vi "globals-engine.vi"() -> ()   [LabVIEW 2024]
uses:
  controls/state-engine.ctl
  controls/type.eng.settings.ctl
  controls/state-logger.ctl
  controls/UiNutritionPanel.ctl
  controls/UiScheduleTimestamp.ctl
  controls/pbr-conf.ctl
  controls/irr-panel.ctl
  controls/enum-com-log.ctl
  controls/enum-q-sched.ctl
panel:
  in  "Q-Sched":refnum<queue>
  out "Q-Com":refnum<queue>
  in  "IRR Params":T1={"Day Time"={"Sunset"=timestamp(0 s since 1904-01-01), "Sunrise"=timestamp(0 s since 1904-01-01)}, "timeLimits"={"Irrigation"=0.0, "Nut./Water"=0.0}, "Calculated Timing"={"Irrigation Timeout"=timestamp(0 s since 1904-01-01), "Nutrients Timeout"=timestamp(0 s since 1904-01-01)}, "Irr Dosing Time"={"Nutrients"=0, "Water"=0, "Wash"=0}, "UV Limit "=0.0, "Dose Table"=[{"Enable"=FALSE, "output"="IRR_SEC1"}, {"Enable"=FALSE, "output"="IRR_SEC2"}, {"Enable"=FALSE, "output"="IRR_SEC3"}, {"Enable"=FALSE, "output"="IRR_SEC4"}, {"Enable"=FALSE, "output"="IRR_SEC5"}, {"Enable"=FALSE, "output"="IRR_SEC6"}], "Last Iteration"=timestamp(0 s since 1904-01-01), "UV Reduction Status"=FALSE, "UV Reduction"=0} {"UV Reduction" max=99 step=1 format="%d [%%]"; "timeLimits"."Nut./Water" format="%02.2f [hr]"; "timeLimits"."Irrigation" format="%02.2f [hr]"; "Day Time"."Sunrise" format="%<%H:%M:%S>T"; "Day Time"."Sunset" format="%<%H:%M:%S>T"; "Calculated Timing"."Nutrients Timeout" format="%<%H:%M:%S>T"; "Calculated Timing"."Irrigation Timeout" format="%<%H:%M:%S>T"; "UV Limit" format="%#.1p [J/m2]"; "Irr Dosing Time"."Wash" format="%d [s]"; "Irr Dosing Time"."Water" format="%d [s]"; "Irr Dosing Time"."Nutrients" format="%d [s]"; "Last Iteration" format="%<%X %x>T"}
  in  "PBRconf":cluster{"units":T2[]} {"units"."Main"."DailyActivityHours"."Begin Time" format="ON:    %<%H:%M>T"; "units"."Main"."DailyActivityHours"."End Time" format="OFF:    %<%H:%M>T"; "units"."Main"."WashTimes"."Out" format="Wash out: %d [sec]"; "units"."Main"."WashTimes"."In" format="Wash in: %d [sec]"}
  in  "NutritionConfiguration":T4[](array[typedef]) {"ORP Dosing"."MIX Limit" format="%d [s]"; "ORP Dosing"."MIX Dose" format="%d [s]"; "PH Dosing"."ACID Limit" format="%d [s]"; "PH Dosing"."BASE Limit" format="%d [s]"; "PH Dosing"."ACID Dose" format="%d [s]"; "PH Dosing"."BASE Dose" format="%d [s]"; "EC Dosing"."BETA2 Limit" format="%d [s]"; "EC Dosing"."ALFA2 Limit" format="%d [s]"; "EC Dosing"."ALFA2 Dose" format="%d [s]"; "EC Dosing"."BETA2 Dose" format="%d [s]"; "EC Dosing"."BETA1 Limit" format="%d [s]"; "EC Dosing"."ALFA1 Limit" format="%d [s]"; "EC Dosing"."ALFA1 Dose" format="%d [s]"; "EC Dosing"."BETA1 Dose" format="%d [s]"; "Main"."DailyActivityHours"."Begin Time" format="ON:    %<%H:%M>T"; "Main"."DailyActivityHours"."End Time" format="OFF:    %<%H:%M>T"; "Main"."WashTimes"."Out" format="Wash out: %d [sec]"; "Main"."WashTimes"."In" format="Wash in: %d [sec]"; "Water Dosing"."Water Limit" format="%d [s]"; "Water Dosing"."Water Dose" format="%d [s]"}
  out "STOP":bool
  in  "Q-Log":refnum<queue>
  in  "NUTRITION_RANGES":T5 {"ALARM"."HIGH" format="%#_13g"; "ALARM"."LOW" format="%#_13g"; "NORMAL"."HIGH" format="%#_13g"; "NORMAL"."LOW" format="%#_13g"}
  in  "ProjectSettings":T6={"Project Name"="Yogiland", "Latitude"=0.0, "Longitude"=0.0, "TimeZone"=0, "userName"="Yogiland"}
  in  "Procedure(pre)":variant[](array[variant])=[variant("procCLK"=variant(dbl 3802946268.2064614), "procIndex"=variant(dbl 2.0), "procIsRunning"=variant(bool TRUE), "procLabel"=variant(string "blink-2"), "procRegisterNumeric"=variant(dbl 3802946266.867457), "procReport"=variant(string "blink-2:3802946268,2>>2,_DELAY_COMPARE,1.3/2.0,STAY"), "procReportPast"=variant(string "blink-2:3802946268,2>>2,_DELAY_COMPARE,1.3/2.0,STAY")), variant("stepFunction"=variant(enum16{"__NO-OP", "_DELAY_LOAD", "_DELAY_COMPARE", "_COMPARE", "_JUMP", "_FINISH", "CLK_COMPARE", "PROC_START", "PROC_STOP", "PROC_ISRUN_COMPARE", "PROC_ISRUN_LOAD", "_IO_READ_IN", "_IO_WRITE_DOUT", "_IO_COMPARE", "Q_OPEN", "Q_WRITE", "Q_READ"} enum."_IO_WRITE_DOUT"), "stepIoPointer"=variant(string "dout2"), "stepIoState(str)"=variant(string "1:1"), "stepLabel"=variant(string "loop"), "stepPath"=variant(string "")), variant("stepFunction"=variant(enum16{"__NO-OP", "_DELAY_LOAD", "_DELAY_COMPARE", "_COMPARE", "_JUMP", "_FINISH", "CLK_COMPARE", "PROC_START", "PROC_STOP", "PROC_ISRUN_COMPARE", "PROC_ISRUN_LOAD", "_IO_READ_IN", "_IO_WRITE_DOUT", "_IO_COMPARE", "Q_OPEN", "Q_WRITE", "Q_READ"} enum."_DELAY_LOAD"), "stepLabel"=variant(string "")), variant("stepFunction"=variant(enum16{"__NO-OP", "_DELAY_LOAD", "_DELAY_COMPARE", "_COMPARE", "_JUMP", "_FINISH", "CLK_COMPARE", "PROC_START", "PROC_STOP", "PROC_ISRUN_COMPARE", "PROC_ISRUN_LOAD", "_IO_READ_IN", "_IO_WRITE_DOUT", "_IO_COMPARE", "Q_OPEN", "Q_WRITE", "Q_READ"} enum."_DELAY_COMPARE"), "stepSetpoint"=variant(cluster{"comparison":string, "Y":dbl} {"comparison"="", "Y"=2.0})), variant("stepFunction"=variant(enum16{"__NO-OP", "_DELAY_LOAD", "_DELAY_COMPARE", "_COMPARE", "_JUMP", "_FINISH", "CLK_COMPARE", "PROC_START", "PROC_STOP", "PROC_ISRUN_COMPARE", "PROC_ISRUN_LOAD", "_IO_READ_IN", "_IO_WRITE_DOUT", "_IO_COMPARE", "Q_OPEN", "Q_WRITE", "Q_READ"} enum."_JUMP"), "stepLabel"=variant(string ""), "stepPointer"=variant(string "loop"))]
  in  "Q-Eng":refnum<queue>
  out "VisaSimulator":bool
  in  "Environment":string
  in  "VISA":refnum<visa-resource-name>
  in  "steps":variant
  in  "stepElemet":variant
  in  "procElement":variant
  # "Water"
  # "EC"
  # "PH"
  # "ORP"
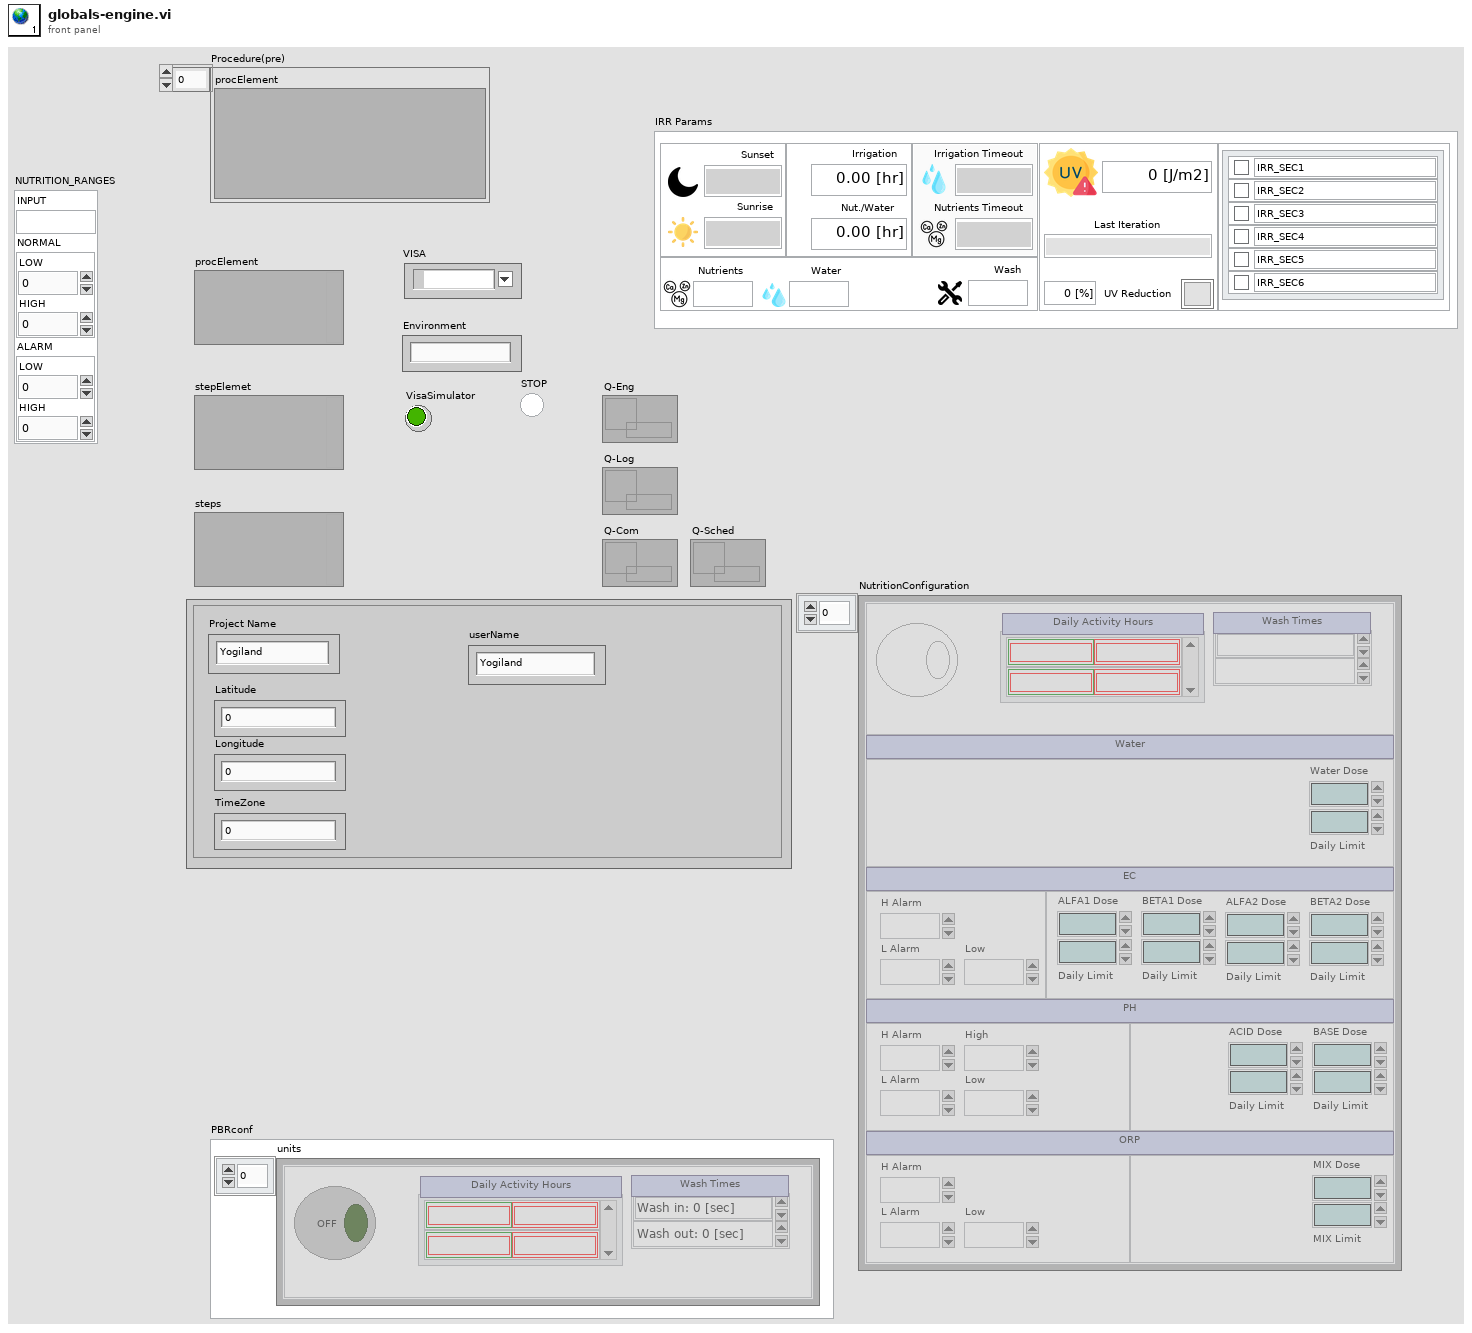
[diagram p1: front panel]
types:
  T1 = typedef "irr-panel.ctl" = cluster{"Day Time":cluster{"Sunset":timestamp, "Sunrise":timestamp}, "timeLimits":cluster{"Irrigation":dbl, "Nut./Water":dbl}, "Calculated Timing":cluster{"Irrigation Timeout":timestamp, "Nutrients Timeout":timestamp}, "Irr Dosing Time":cluster{"Nutrients":u16, "Water":u16, "Wash":u16}, "UV Limit ":dbl, "Dose Table":cluster{"Enable":bool, "output":string}[], "Last Iteration":timestamp, "UV Reduction Status":bool, "UV Reduction":u8}
  T2 = typedef "pbr-conf.ctl" = cluster{"Main":cluster{"Enable":bool, "WashTimes":cluster{"In":dbl, "Out":dbl}, "DailyActivityHours":cluster{"Begin Time":T3, "End Time":T3}[]}}
  T3 = typedef "UiScheduleTimestamp.ctl" = timestamp
  T4 = typedef "UiNutritionPanel.ctl" = cluster{"Main":cluster{"Enable":bool, "WashTimes":cluster{"In":dbl, "Out":dbl}, "DailyActivityHours":cluster{"Begin Time":T3, "End Time":T3}[]}, "Water Dosing":cluster{"Water Dose":dbl, "Water Limit":dbl}, "EC Ranges":cluster{"H Alarm":dbl, "L Alarm":dbl, "Low":dbl}, "EC Dosing":cluster{"ALFA1 Dose":dbl, "ALFA1 Limit":dbl, "BETA1 Dose":dbl, "BETA1 Limit":dbl, "ALFA2 Dose":dbl, "ALFA2 Limit":dbl, "BETA2 Dose":dbl, "BETA2 Limit":dbl}, "PH Ranges":cluster{"H Alarm":dbl, "L Alarm":dbl, "High":dbl, "Low":dbl}, "PH Dosing":cluster{"ACID Dose":dbl, "ACID Limit":dbl, "BASE Dose":dbl, "BASE Limit":dbl}, "ORP Ranges":cluster{"H Alarm":dbl, "L Alarm":dbl, "Low":dbl}, "ORP Dosing":cluster{"MIX Dose":dbl, "MIX Limit":dbl}}
  T5 = cluster{"INPUT":string, "NORMAL":cluster{"LOW":dbl, "HIGH":dbl}, "ALARM":cluster{"LOW":dbl, "HIGH":dbl}}
  T6 = typedef "type.eng.settings.ctl" = cluster{"Project Name":string, "Latitude":dbl, "Longitude":dbl, "TimeZone":i32, "userName":string}
diagram:
